vi "_Create Queue.vi"(9 "Queue jettl":refnum<class "Queue jettl.lvclass">, 10 "Alias":string) -> (3 "Create Queue Msg Strategy out":refnum<class "Create Queue Msg Strategy.lvclass">)   [LabVIEW 2021, in "jettl Msg Create Queue.lvlib"]
uses:
  jettl Msg Create Queue.lvlib
  Create Queue Msg Strategy/Create Queue Msg Strategy.lvclass
  jettl/Queue jettl/Queue jettl.lvclass
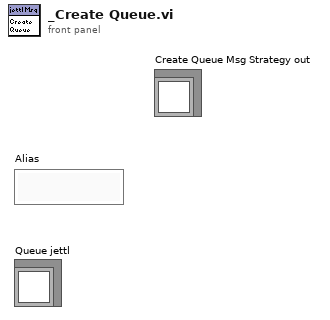
[diagram p1: front panel]
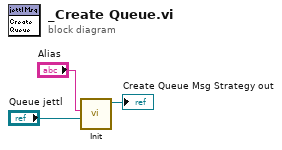
[diagram p0: block diagram]
diagram:
  n1 = call "Init.vi"("Queue jettl"="Queue jettl", "Alias"="Alias") -> ("Create Queue Msg Strategy out"=→"Create Queue Msg Strategy out":refnum<class "Create Queue Msg Strategy.lvclass">)  [unwired: 9 in]
